vi "observacao.vi"() -> ()   [LabVIEW 2018, in "Shared_160.lvlib"] (continued)
            n314 = Select(t=FALSE, s=w274, f=w271) -> (s? t:f=w273:bool)
            n315 = case shown="False" w276 {
              frame False {
                w313 = 0
                n316 = property on="BtPointPrecess" class="Bool"("DisabledEnum"=w313) -> ()  [unwired: 2 in, 2 out]
                n317 = property on="BtPointObjClear" class="Bool"("DisabledEnum"=w313) -> ()  [unwired: 2 in, 2 out]
              }
              frame True {
                w314 = 2
                n318 = property on="BtPointPrecess" class="Bool"("DisabledEnum"=w314) -> ()  [unwired: 2 in, 2 out]
                n319 = property on="BtPointObjClear" class="Bool"("DisabledEnum"=w314) -> ()  [unwired: 2 in, 2 out]
              }
            }
            n320 = case shown="True" w273 {
              tunnel: [w384 w401] -> w299
              tunnel: [w383 w400] -> w295
              tunnel: [w386 w404] -> w275
              tunnel: [w385 w402] -> w292
              tunnel: w307 -> [w384 w401]
              tunnel: w306 -> [w389 _]
              tunnel: w305 -> [w388 _]
              tunnel: w302 -> [w387 _]
              tunnel: [w382 w398] -> _
              tunnel: w269 -> [w382 w398]
              frame False {
                n321 = case shown="True" w387 {
                  tunnel: w388 -> [w391 w397]
                  tunnel: [w391 w396] -> w386
                  tunnel: w389 -> [w390 w395]
                  tunnel: [w390 w392] -> w385
                  frame False {
                  }
                  frame True {
                    n322 = global read "Global_Telescopio.vi" "Calagem AH"() -> (w393:dbl)
                    n323 = global read "Global_Telescopio.vi" "Calagem DEC"() -> (w394:dbl)
                    n324 = Subtract(x=w395, y=w393) -> (x-y=w392:dbl)
                    n325 = Subtract(x=w397, y=w394) -> (x-y=w396:dbl)
                  }
                }
                n326 = Subtract(x=w384, y=w385) -> (x-y=w383:dbl)
              }
              frame True {
                # "PROCESSO PRECESSÃO"
                n327 = local read "Temp amb"() -> (w407:string)
                n328 = local read "hum local"() -> (w405:string)
                n329 = local read "MeanDEC"() -> (w408:string)
                n330 = local read "pressão atm"() -> (w406:string)
                n331 = local read "PM_RA"() -> (w403:string)
                n332 = local read "MeanRA"() -> (w409:string)
                n333 = local read "PM_DEC"() -> (w399:string)
                n334 = call "PrecessFortran.vi"("Asc reta"=w409, "Var RA"=w403, "Declinação"=w408, "Temperatura (Kelvin)"=w407, "Pressao atmosferica (mB)"=w406, "Humidade relativa (0 a 1)"=w405, "Var DEC"=w399) -> ("Observed RA (radians)"=w400:dbl, "Observed Dec (radians)"=w404:dbl)  [unwired: 2 in, 5 out]
                n335 = Subtract(x=w401, y=w400) -> (x-y=w402:dbl)
              }
            }
            "AtualDEC" <- w275
            n336 = case shown="True" w273 {
              tunnel: [w335 w338] -> w304
              tunnel: [w335 w337] -> w303
              tunnel: w275 -> [_ w336]
              frame False {
                w335 = 0.0
              }
              frame True {
                n337 = stacked-sequence {
                  seq-local: [w339 _ _] -> [_ _ w377]
                  tunnel: [_ w346 _] -> w338
                  tunnel: [_ w345 _] -> w337
                  tunnel: w336 -> [_ w340 _]
                  frame #0 {
                    n338 = Tick Count (ms)() -> (millisecond timer value=w339:u32)
                  }
                  frame #1 {
                    w347 = u16 3 items=["Alarme", "Atencao", "Erro", "Ocupado", "Protecao", "Embreagem", "Tracking", "Var. Track", "Rápido", "Ligeiro", "Médio", "Lento", "Em movimento", ""] ("NomeStatus")
                    w348 = u16 3 items=["Alarme", "Atencao", "Erro", "Ocupado", "Protecao", "Embreagem", "Tracking", "Var. Track", "Rápido", "Ligeiro", "Médio", "Lento", "Em movimento", ""] ("NomeStatus")
                    # "PROCESSO LEITURA POS_MOTOR"
                    n339 = local read "MOV_IDX_AH"() -> (w343:bool)
                    n340 = local read "MOV_IDX_DEC"() -> (w341:bool)
                    n341 = call "Bit Status AH.vi"("NomeStatus"=w348) -> ("StatBit"=w344:bool)
                    n342 = call "Bit Status DEC.vi"("NomeStatus"=w347) -> ("StatBit"=w342:bool)
                    n343 = case shown="False" w344 {
                      tunnel: w340 -> [w362 _]
                      tunnel: [w361 w376] -> w346
                      tunnel: w343 -> [w360 _]
                      frame False {
                        n344 = case shown="False" w360 {
                          tunnel: w362 -> [w370 _]
                          tunnel: [w366 w375] -> w361
                          frame False {
                            w373 = u16 1 items=["ZERO", "AH", "DEC", "TUBO", "CUP"] ("Controlador")
                            # "RA"
                            # "AH"
                            n345 = call "Get Posic Motor Indexer.vi"("Controlador"=w373) -> ("PosMotor"=w364:dbl)
                            n346 = global read "Global_Telescopio.vi" "AcumPrecRA"() -> (w367:dbl)
                            n347 = Negate(x=w364) -> (-x=w365:dbl)
                            n348 = Subtract(x=w365, y=w367) -> (x-y=w374:dbl)
                            n349 = global read "Global_Telescopio.vi" "AcumAG RA"() -> (w368:dbl)
                            n350 = Cosine(x=w370) -> (cos(x)=w369:dbl)
                            n351 = Absolute Value(x=w369) -> (abs(x)=w363:dbl)
                            n352 = Subtract(x=w374, y=w368) -> (x-y=w372:dbl)
                            n353 = Multiply(x=w363, y=w372) -> (x*y=w371:dbl)
                            n354 = call "Rad to Arcsec.vi"("Radiano"=w371) -> ("Arcsec"=w366:dbl)
                          }
                          frame True {
                            n355 = local read "Offset RA"() -> (w375:dbl)
                          }
                        }
                      }
                      frame True {
                        n356 = local read "Offset RA"() -> (w376:dbl)
                      }
                    }
                    n357 = case shown="False" w342 {
                      tunnel: [w350 w359] -> w345
                      tunnel: w341 -> [w349 _]
                      frame False {
                        n358 = case shown="False" w349 {
                          tunnel: [w351 w358] -> w350
                          frame False {
                            w354 = u16 2 items=["ZERO", "AH", "DEC", "TUBO", "CUP"] ("Controlador")
                            n359 = call "Get Posic Motor Indexer.vi"("Controlador"=w354) -> ("PosMotor"=w356:dbl)
                            n360 = global read "Global_Telescopio.vi" "AcumPrecDEC"() -> (w352:dbl)
                            n361 = Subtract(x=w356, y=w352) -> (x-y=w357:dbl)
                            n362 = global read "Global_Telescopio.vi" "AcumAG DEC"() -> (w353:dbl)
                            n363 = Subtract(x=w357, y=w353) -> (x-y=w355:dbl)
                            n364 = call "Rad to Arcsec.vi"("Radiano"=w355) -> ("Arcsec"=w351:dbl)
                          }
                          frame True {
                            n365 = local read "Offset DEC"() -> (w358:dbl)
                          }
                        }
                      }
                      frame True {
                        n366 = local read "Offset DEC"() -> (w359:dbl)
                      }
                    }
                  }
                  frame #2 {
                    n367 = flat-sequence {
                      tunnel: w377 -> [w378]
                      frame #0 {
                        n368 = Tick Count (ms)() -> (millisecond timer value=w379:u32)
                        n369 = Subtract(x=w379, y=w379) -> (x-y=→"dtAUX2":u32)
                        n370 = Subtract(x=w379, y=w378) -> (x-y=→"dtAUX3":u32)
                      }
                    }
                  }
                }
              }
            }
            "Offset RA" <- w304
            "Offset DEC" <- w303
            n371 = Add(x=w297, y=w295) -> (x+y=w296:dbl)
            n372 = Add(x=w297, y=w299) -> (x+y=w300:dbl)
            n373 = Less Than 0?(x=w299) -> (x < 0?=w301:bool)
            n374 = Less Than 0?(x=w295) -> (x < 0?=w298:bool)
            n375 = call "Normliza_AH.vi"("PosAH"=w292) -> ("Numeric"=w279:dbl)
            n376 = Select(t=w300, s=w301, f=w299) -> (s? t:f=w280:dbl)
            n377 = Select(t=w296, s=w298, f=w295) -> (s? t:f=w281:dbl)
            n378 = case shown="True" w271 {
              tunnel: ["" w322] -> w282
              tunnel: w281 -> [_ w319]
              tunnel: w280 -> [_ w320]
              tunnel: w275 -> [_ w321]
              frame False {
              }
              frame True {
                n379 = disable-structure shown="Disabled" {
                  disable-tunnel: w321 -> [w333 _]
                  disable-tunnel: w320 -> [w332 _]
                  disable-tunnel: w319 -> [w331 _]
                  disable-tunnel: [w330 _] -> _
                  frame Disabled {
                    n380 = call "Hora_Limite.vi"("Asc Reta RA rad"=w331, "Sideral Time rad"=w332, "Declinação rad"=w333) -> ("TO Tempo de Observação Horas"=w330:dbl)  [unwired: 2 in]
                  }
                  frame Enabled {
                  }
                }
                n381 = call "Novo_tempo_obs.vi"() -> ("TO rad"=w317:dbl)  [unwired: 10 in, 1 out]
                n382 = Greater Than 0?(x=w317) -> (x > 0?=w316:bool)
                n383 = case shown="True" w316 {
                  tunnel: [w324 w327] -> w318
                  tunnel: w317 -> [w324 w326]
                  frame False {
                  }
                  frame True {
                    n384 = Random Number (0-1)() -> (number: 0 to 1=w328:dbl)
                    n385 = Multiply(x=w328, y=7.27e-05) -> (x*y=w325:dbl)
                    n386 = Add(x=w326, y=w325) -> (x+y=w327:dbl)
                  }
                }
                n387 = call "rad_hms.vi"("TRUE=HORA\nFALSE=GRAU"=TRUE ("TRUE=HORA\nFALSE=GRAU"), "Radiano"=w318) -> ("Hora/Graus Texto Decimal"=w322:string)  [unwired: 3 in]
              }
            }
            "Time to Limit" <- w282
            n388 = global write "Global_Telescopio.vi" "AH_now"(w279) -> ()
            n389 = call "rad_hms.vi"("TRUE=HORA\nFALSE=GRAU"=TRUE ("TRUE=HORA\nFALSE=GRAU"), "Radiano"=w280) -> ("Hora/Graus Texto Decimal"=w294:string)  [unwired: 3 in]
            "Sideral time" <- w294
            n390 = call "rad_hms.vi"("TRUE=HORA\nFALSE=GRAU"=TRUE, "Radiano"=w281) -> ("Hora/Graus Texto Decimal"=w293:string)  [unwired: 3 in]
            "Right Ascention" <- w293
            n391 = call "rad_hms.vi"("TRUE=HORA\nFALSE=GRAU"=TRUE, "Radiano"=w279) -> ("Hora/Graus Texto Decimal"=w278:string)  [unwired: 3 in]
            "Hour Angle" <- w278
            "Hour Angle 2" <- w278
            n392 = call "rad_hms.vi"("TRUE=HORA\nFALSE=GRAU"=FALSE, "Radiano"=w275) -> ("Hora/Graus Texto Decimal"=w277:string)  [unwired: 3 in]
            "Declination" <- w277
            "DEC" <- w277
            n393 = global write "Global_Telescopio.vi" "Right Ascention"(w293) -> ()
            n394 = global write "Global_Telescopio.vi" "Hour Angle"(w278) -> ()
            n395 = global write "Global_Telescopio.vi" "Sideral time"(w294) -> ()
            n396 = global write "Global_Telescopio.vi" "Declination"(w277) -> ()
            n397 = global write "Global_Telescopio.vi" "delta_now"(w275) -> ()
          }
          frame #2 {
            w433 = -0.39330025  # LatOPD rad
            # "ALTERAÇÃO FEITA EM 12/12/2012\nFEITA PARA RESOLVER EXCESSÍVOS\nMOVIMENTOS DO ACOMP.SID. DA\nCÚPULA (DANIEL). A condição de statCUP=0 foi inserida em 08/5/2013-> Só corrige a cúpula se esta estiver parada!"
            # "Horas"
            # "MUDANÇA FUTURA:\nPassar LatOPD para Global"
            # "az"
            # "z"
            # "Cálculo do Azimute da Cúpula e Hab Acompanham. Cúpula"
            # "Lógica de Segurança"
            # "ANGULO ZENITAL"
            n398 = global read "Global_Telescopio.vi" "OffsetCupula"() -> (w442:dbl)
            n399 = global read "Global_Telescopio.vi" "AH_now"() -> (w425:dbl)
            n400 = global read "Global_Telescopio.vi" "delta_now"() -> (w432:dbl)
            n401 = global read "Global_Telescopio.vi" "Limite EAST"() -> (w426:dbl)
            n402 = global read "Global_Telescopio.vi" "Limite WEST"() -> (w427:dbl)
            n403 = call "Calculo_do_Azimute_da_Cupula_2.vi"("AH"=w425, "DEC"=w432, "OffsetTCSPD"=w442) -> ("PosCup"=w411:u16)  [unwired: 3 in, 1 out]
            "Azimute cup" <- w411
            n404 = local read "Tick Cupula"() -> (w417:u32)
            n405 = Tick Count (ms)() -> (millisecond timer value=w418:u32)
            n406 = global read "Global_Telescopio.vi" "PosCUP"() -> (→"PosCUP":i16)
            n407 = Multiply(x=w425, y=3.8197) -> (x*y=w428:dbl)
            n408 = call "Altura_e_Azimute.vi"("LAT rad"=w433, "DEC rad"=w432, "AH rad"=w425) -> ("AZIMUTE graus"=w413:dbl, "ANG. ZENITAL graus"=w431:dbl, "AZIMUTE rad"=w434:dbl, "ANG. ZENITAL rad"=w435:dbl)  [unwired: 2 out]
            "Azimuth" <- w413
            "Zenital angle" <- w431
            n409 = Greater Or Equal?(x=w418, y=w417) -> (x >= y?=w416:bool)
            n410 = Greater?(x=w428, y=w426) -> (0:w424:bool)
            n411 = Less?(x=w428, y=w427) -> (x < y?=w423:bool)
            n412 = call "Checa destino cupula.vi"("Target"=w411) -> ("moverCup"=w410:bool)  [unwired: 6 in, 2 out]
            n413 = local read "statCUP"() -> (w415:i32)
            n414 = Not And(1:w423, 2:w424) -> (0:w420:bool)
            n415 = Equal To 0?(x=w415) -> (x = 0?=w414:bool)
            n416 = call "Calcula_Proteção.vi"("Zenital angle rad"=w435, "Azimute rad"=w434) -> ("Z_SEGURANÇA_GRAUS"=w444:dbl, "Prot Segur"=w446:bool, "Z_LIBERA_GRAUS"=w443:dbl, "Z_MAX_GRAUS"=w445:dbl, "Prot Zmax"=w421:bool)
            n417 = Compound Arithmetic op=AND(w410, "DOME", w416, w414) -> (w441:bool)
            n418 = case shown="True" w441 {
              tunnel: w411 -> [_ w450]
              tunnel: FALSE -> [_ w455]
              frame False {
              }
              frame True {
                # "TEMPO CÚPULA"
                # "2m Tempo para novo movimento"
                n419 = Tick Count (ms)() -> (millisecond timer value=w454:u32)
                n420 = local write "Dome on Target"(w455) -> ()
                n421 = To Word Integer(number=w450) -> (16bit integer=w451:i16)
                n422 = Add(x=w454, y=u32 120000) -> (x+y=→"Tick Cupula":u32)
                n423 = local write "statCUP"(1 ("statCUP")) -> ()
                n424 = Number To Decimal String(number=w450) -> (decimal integer string=→"TargetCup":string)  [unwired: 1 in]
                n425 = global write "Global_Telescopio.vi" "TargetCUP"(w451) -> ()
              }
            }
            n426 = global write "Global_Telescopio.vi" "Z_SEGURANÇA_GRAUS"(w444) -> ()
            n427 = global write "Global_Telescopio.vi" "Zenital angle GRAUS"(w431) -> ()
            n428 = global write "Global_Telescopio.vi" "Azimute GRAUS"(w413) -> ()
            n429 = global write "Global_Telescopio.vi" "Z_MAX_GRAUS"(w445) -> ()
            n430 = global write "Global_Telescopio.vi" "Z_LIBERA_GRAUS"(w443) -> ()
            n431 = global read "Global_Telescopio.vi" "LIMITE"() -> (w440:bool)
            n432 = Or(x=w420, y=w421) -> (x .or. y?=w422:bool)
            n433 = Or(x=w440, y=w422) -> (x .or. y?=w439:bool)
            "Proteção" <- w439
            n434 = call "Borda_Subida_Z_max.vi"("Entrada"=w439) -> ("Boolean"=w448:bool)
            n435 = call "Borda_Subida_Segurança.vi"("Entrada"=w446) -> ("Boolean"=w447:bool)
            n436 = case shown="True" w448 {
              frame False {
              }
              frame True {
                w463 = FALSE
                w461 = "Telescópio parado por inclinação excessiva!" ("SYSTEM MESSAGES")
                n437 = local write "LED MOUNT"(w463) -> ()
                n438 = local write "MOUNT"(w463) -> ()
                n439 = global write "Global_Telescopio.vi" "ObjCentrado"(FALSE) -> ()
                n440 = global write "Global_Telescopio.vi" "STOP ALL"(TRUE ("STOP ALL")) -> ()
                n441 = call "Monta_Mensagem.vi"("Mensagem"=w461) -> ()  [unwired: 2 in]
                n442 = call "Salva_systems_messages.vi"("Mensagem"=w461) -> ()  [unwired: 5 in]
              }
            }
            n443 = Select(t=u8 2 ("Disabled"), s=w439, f=u8 0 ("Disabled")) -> (s? t:f=w436:u8)
            n444 = case shown="True" w447 {
              frame False {
              }
              frame True {
                w459 = u16 2 items=["ZERO", "AH", "DEC", "TUBO", "CUP"] ("Controlador")
                w458 = "FREAR" ("Comando")
                w460 = u16 1 items=["ZERO", "AH", "DEC", "TUBO", "CUP"] ("Controlador")
                w457 = "EIXO" ("Dispositivo")
                n445 = call "Monta Comando.vi"("Comando"=w458, "Dispositivo"=w457, "Controlador"=w460) -> ()  [unwired: 2 in, 5 out]
                n446 = call "Monta Comando.vi"("Comando"=w458, "Dispositivo"=w457, "Controlador"=w459) -> ()  [unwired: 2 in, 5 out]
              }
            }
            n447 = property on="MOUNT" class="Bool (strict)"("Disabled"=w436) -> ()  [unwired: 2 in, 2 out]
            "Led Chave Dome" <- "DOME"
          }
          frame #3 {
            w470 = u32 500 ("millisecond multiple")
            w484 = u16 3 items=["Alarme", "Atencao", "Erro", "Ocupado", "TBD", "LCB", "Trapeira", "Paravento", "DomoRap", "DomoCW", "DomoCCW", "TBD", "Em movimento", "TBD"] ("NomeStatus")
            w496 = u16 3 items=["Alarme", "Atencao", "Erro", "Ocupado", "Protecao", "Embreagem", "Tracking", "Var. Track", "Rápido", "Ligeiro", "Médio", "Lento", "Em movimento", ""] ("NomeStatus")
            w497 = u16 3 items=["Alarme", "Atencao", "Erro", "Ocupado", "Protecao", "Embreagem", "Tracking", "Var. Track", "Rápido", "Ligeiro", "Médio", "Lento", "Em movimento", ""] ("NomeStatus")
            # "04-07-2022\nValor de Erro PROTEC\nalterado de 5 para 10"
            # "MUDANÇA: \nIncluído CASE"
            # "Esse metrônomo determina\no ciclo de 0,5 segundo dos\ncálculos rápidos e totais!"
            # "PROCESSO APONTAMENTO"
            # "MÁQUINA DE ESTADO DO APONTAMENTO"
            # "Seta nome para GO/STOP"
            n448 = global read "Global_Telescopio.vi" "PosDEC"() -> (w499:dbl)
            n449 = global read "Global_Telescopio.vi" "TargetDEC"() -> (w500:dbl)
            n450 = global read "Global_Telescopio.vi" "LimiarRapMed"() -> (w498:dbl)
            n451 = global read "Global_Telescopio.vi" "ErroMaxEixo"() -> (w487:dbl)
            n452 = call "Bit Status DEC.vi"("NomeStatus"=w496) -> ("StatBit"=w486:bool)
            n453 = global read "Global_Telescopio.vi" "Sideral Time"() -> (w478:dbl)
            n454 = global read "Global_Telescopio.vi" "PosAH"() -> (w501:dbl)
            n455 = global read "Global_Telescopio.vi" "TargetRA"() -> (w502:dbl)
            n456 = global write "Global_Telescopio.vi" "Estado AH"("statAH") -> ()
            n457 = call "Bit Status AH.vi"("NomeStatus"=w497) -> ("StatBit"=w485:bool)
            n458 = case shown="40" "statDEC" {
              selector: "statDEC" -> [w631 _ _ _ _ _ _ _ _]
              tunnel: [w631 w638 w668 w690 w717 w741 0 ("t") w758 w768] -> w479
              tunnel: w500 -> [_ w637 _ w684 _ _ _ _ w774]
              tunnel: w499 -> [_ w633 _ w687 _ _ _ _ w773]
              tunnel: w487 -> [_ _ _ w688 _ _ _ _ w771]
              tunnel: w498 -> [_ w639 _ _ _ _ _ _ _]
              tunnel: w486 -> [_ w636 _ w683 _ _ _ _ _]
              frame 0, Default {
                w629 = 0 ("CR DEC")
                # "Sem apontamento"
                n459 = call "TickTimeout.vi"() -> ("msTick"=→"TimeoutDEC":u32)  [unwired: 2 in, 2 out]
                n460 = local write "CR DEC"(w629) -> ()
                n461 = local write "C. DEC"(w629) -> ()
              }
              frame 1 {
                # "Envia\nComando"
                n462 = Subtract(x=w637, y=w633) -> (x-y=w635:dbl)
                n463 = Absolute Value(x=w635) -> (abs(x)=w640:dbl)
                n464 = local write "dec="(FALSE ("dec=")) -> ()
                n465 = Less?(x=w640, y=w639) -> (x < y?=w634:bool)
                n466 = case shown="False" w634 {
                  tunnel: [w644 3] -> w638
                  tunnel: w637 -> [w643 _]
                  tunnel: w635 -> [w642 _]
                  tunnel: w636 -> [w641 _]
                  frame False {
                    # "destino"
                    # "Fora do"
                    n467 = case shown="False" w641 {
                      tunnel: [w648 w656] -> w644
                      tunnel: w643 -> [w651 _]
                      tunnel: w642 -> [_ _]
                      frame False {
                        w655 = u16 2 items=["ZERO", "AH", "DEC", "TUBO", "CUP"] ("Controlador")
                        # "limpa flag"
                        # "CLP Pronto"
                        n468 = local write "Flag ativo DEC"(FALSE ("Flag ativo DEC")) -> ()
                        n469 = call "rad_hms.vi"("TRUE=HORA\nFALSE=GRAU"=FALSE, "Radiano"=w651) -> ("Hora/Graus Texto Decimal"=w652:string)  [unwired: 3 in]
                        n470 = call "Monta Comando.vi"("Set Point"=w652, "Comando"="MOVER_RAP", "Dispositivo"="EIXO" ("Comando"), "Controlador"=w655) -> ("Erro Comunicação"=w646:bool)  [unwired: 1 in, 4 out]
                        n471 = Select(t=6, s=w646, f=20) -> (s? t:f=w648:i32)
                      }
                      frame True {
                        # "CLP Ocupado"
                        n472 = local read "TimeoutDEC"() -> (w658:u32)
                        n473 = call "TickTimeout.vi"("msInicial"=w658, "msTimeout"=u32 4000) -> ("Timeout"=w657:bool)  [unwired: 2 out]
                        n474 = case shown="False" w657 {
                          tunnel: [1 5] -> w656
                          frame False {
                          }
                          frame True {
                            # "Tratar\nTimeout"
                          }
                        }
                      }
                    }
                  }
                  frame True {
                    # "Dist. pequena p/ mov. rápido"
                    # "Ligar mov. lento"
                    n475 = call "TickTimeout.vi"() -> ("msTick"=w662:u32)  [unwired: 2 in, 2 out]
                    n476 = local write "TimeoutDEC"(w662) -> ()
                  }
                }
              }
              frame 2 {
                w669 = u16 12 items=["Alarme", "Atencao", "Erro", "Ocupado", "Protecao", "Embreagem", "Tracking", "Var. Track", "Rápido", "Ligeiro", "Médio", "Lento", "Em movimento", ""] ("NomeStatus")
                # "Aguarda fim mov. Rap."
                n477 = global read "Global_Telescopio.vi" "Habilita supervisao"() -> (w665:bool)
                n478 = call "Bit Status DEC.vi"("NomeStatus"=w669) -> ("StatBit"=w670:bool)
                n479 = case shown="True" w670 {
                  tunnel: [1 w679] -> w667
                  frame False {
                    # "Motor parado.\nTestar se chegou\nao destino"
                    n480 = call "TickTimeout.vi"() -> ("msTick"=w675:u32)  [unwired: 2 in, 2 out]
                    n481 = local write "TimeoutDEC"(w675) -> ()
                  }
                  frame True {
                    # "Ainda movendo...\nAGUARDAR"
                    n482 = local read "Erro PROTEC"() -> (w681:i32)
                    n483 = call "PROTECAO_DEC.vi"() -> ("CONT DEC"=w682:i32)  [unwired: 11 in]
                    "C. DEC" <- w682
                    n484 = Greater Or Equal?(x=w682, y=w681) -> (x >= y?=w677:bool)
                    n485 = Select(t=6, s=w677, f=2) -> (s? t:f=w679:i32)
                  }
                }
                n486 = case shown="False" w665 {
                  tunnel: [FALSE w674] -> w664
                  frame False {
                  }
                  frame True {
                    n487 = local read "Erro Lim"() -> (w672:i32)
                    n488 = Greater Or Equal?(x="CR DEC", y=w672) -> (x >= y?=w674:bool)
                  }
                }
                n489 = Select(t=6, s=w664, f=w667) -> (s? t:f=w668:i32)
              }
              frame 3 {
                # "Mov.Lento"
                n490 = Subtract(x=w684, y=w687) -> (x-y=w685:dbl)
                n491 = Absolute Value(x=w685) -> (abs(x)=w689:dbl)
                n492 = Less Or Equal?(x=w689, y=w688) -> (x <= y?=w686:bool)
                n493 = case shown="False" w686 {
                  selector: w686 -> [_ w713]
                  tunnel: [w692 0] -> w690
                  tunnel: w685 -> [w691 _]
                  tunnel: w684 -> [_ w712]
                  tunnel: w683 -> [w693 _]
                  frame False {
                    n494 = case shown="False" w693 {
                      tunnel: [w697 w706] -> w692
                      tunnel: w691 -> [w700 _]
                      frame False {
                        w705 = u16 2 items=["ZERO", "AH", "DEC", "TUBO", "CUP"] ("Controlador")
                        # "limpa flag"
                        # "Mov. lento"
                        n495 = call "rad_hms.vi"("TRUE=HORA\nFALSE=GRAU"=FALSE ("TRUE=HORA\nFALSE=GRAU"), "Radiano"=w700) -> ("Hora/Graus Texto Decimal"=w702:string)  [unwired: 3 in]
                        n496 = call "Monta Comando.vi"("Set Point"=w702, "Comando"="MOVER_REL", "Dispositivo"="EIXO" ("Comando"), "Controlador"=w705) -> ("Erro Comunicação"=w695:bool)  [unwired: 1 in, 4 out]
                        n497 = call "TickTimeout.vi"() -> ("msTick"=w699:u32)  [unwired: 2 in, 2 out]
                        n498 = local write "Flag ativo DEC"(FALSE ("Flag ativo DEC")) -> ()
                        n499 = local write "TimeoutDEC"(w699) -> ()
                        n500 = Select(t=6, s=w695, f=40) -> (s? t:f=w697:i32)
                      }
                      frame True {
                        # "CLP Ocupado"
                        n501 = local read "TimeoutDEC"() -> (w708:u32)
                        n502 = call "TickTimeout.vi"("msInicial"=w708, "msTimeout"=u32 2000) -> ("Timeout"=w707:bool)  [unwired: 2 out]
                        n503 = case shown="False" w707 {
                          tunnel: [3 5] -> w706
                          frame False {
                          }
                          frame True {
                          }
                        }
                      }
                    }
                  }
                  frame True {
                    # "DEC no destino"
                    n504 = local write "LatchDeslocDEC"(w712) -> ()
                    "DEC on Target" <- w713
                  }
                }
              }
              frame 4 {
                w720 = u16 12 items=["Alarme", "Atencao", "Erro", "Ocupado", "Protecao", "Embreagem", "Tracking", "Var. Track", "Rápido", "Ligeiro", "Médio", "Lento", "Em movimento", ""] ("NomeStatus")
                # "Aguarda fim mov. lento"
                n505 = global read "Global_Telescopio.vi" "Habilita supervisao"() -> (w718:bool)
                n506 = call "Bit Status DEC.vi"("NomeStatus"=w720) -> ("StatBit"=w721:bool)
                n507 = case shown="False" w721 {
                  tunnel: [3 w731] -> w716
                  frame False {
                    # "Motor parado.\nTestar se chegou\nao destino"
                    n508 = call "TickTimeout.vi"() -> ("msTick"=w726:u32)  [unwired: 2 in, 2 out]
                    n509 = local write "TimeoutDEC"(w726) -> ()
                  }
                  frame True {
                    n510 = local read "Erro PROTEC"() -> (w733:i32)
                    n511 = call "PROTECAO_DEC.vi"() -> ("CONT DEC"=w728:i32)  [unwired: 11 in]
                    n512 = local write "C. DEC"(w728) -> ()
                    n513 = Greater Or Equal?(x=w728, y=w733) -> (x >= y?=w730:bool)
                    n514 = local read "TimeoutDEC"() -> (w735:u32)
                    n515 = call "TickTimeout.vi"("msInicial"=w735, "msTimeout"=u32 4000) -> ("Timeout"=w734:bool)  [unwired: 2 out]
                    n516 = case shown="False" w734 {
                      tunnel: [4 5] -> w729
                      frame False {
                      }
                      frame True {
                      }
                    }
                    n517 = Select(t=6, s=w730, f=w729) -> (s? t:f=w731:i32)
                  }
                }
                n518 = case shown="True" w718 {
                  tunnel: [FALSE w725] -> w715
                  frame False {
                  }
                  frame True {
                    n519 = local read "CR DEC"() -> (w724:i32)
                    n520 = local read "Erro Lim"() -> (w723:i32)
                    n521 = Greater Or Equal?(x=w724, y=w723) -> (x >= y?=w725:bool)
                  }
                }
                n522 = Select(t=6, s=w715, f=w716) -> (s? t:f=w717:i32)
              }
              frame 5 {
                w746 = u16 2 items=["ZERO", "AH", "DEC", "TUBO", "CUP"] ("Controlador")
                # "Reiniciar apontamento"
                # "Trata Timeout"
                n523 = call "TickTimeout.vi"() -> ("msTick"=w743:u32)  [unwired: 2 in, 2 out]
                n524 = local write "TimeoutDEC"(w743) -> ()
                n525 = call "Monta Comando.vi"("Comando"="PARAR", "Dispositivo"="PROG" ("Comando"), "Controlador"=w746) -> ("Erro Comunicação"=w739:bool)  [unwired: 2 in, 4 out]
                n526 = Select(t=6, s=w739, f=1) -> (s? t:f=w741:i32)
              }
              frame 6 {
                # "PARADA POR ERRO DO CONTROLADOR"
                n527 = stacked-sequence {
                  frame #0 {
                    w749 = u16 2 items=["ZERO", "AH", "DEC", "TUBO", "CUP"] ("Controlador")
                    n528 = call "Monta Comando.vi"("Comando"="PARAR", "Dispositivo"="PROG" ("Comando"), "Controlador"=w749) -> ()  [unwired: 2 in, 5 out]
                    "dec=" <- TRUE ("ah=")
                  }
                  frame #1 {
                    w752 = "Erro de Controlador DEC , REAPONTAR !" ("Mensagem")
                    n529 = local write "Flag de erro p/ apagar lampada"(TRUE ("Flag de erro p/ apagar lampada")) -> ()
                    n530 = call "Monta_Mensagem.vi"("Mensagem"=w752) -> ()  [unwired: 2 in]
                    n531 = call "Salva_systems_messages.vi"("Mensagem"=w752) -> ()  [unwired: 5 in]
                  }
                  frame #2 {
                    w755 = u16 2 items=["ZERO", "AH", "DEC", "TUBO", "CUP"] ("Controlador")
                    # "Em movimento não aceita reset"
                    # "Segundo PARAR por garantia"
                    n532 = call "Monta Comando.vi"("Comando"="PARAR", "Dispositivo"="PROG", "Controlador"=w755) -> ()  [unwired: 2 in, 5 out]
                  }
                }
              }
              frame 20 {
                # "Espera entrar\nem movimento"
                n533 = local read "Flag ativo DEC"() -> (w757:bool)
                n534 = case shown="True" w757 {
                  tunnel: [20 ("t") 2 ("t")] -> w758
                  frame False {
                  }
                  frame True {
                    # "limpa flag"
                    n535 = local write "Flag ativo DEC"(FALSE ("Flag ativo AH")) -> ()
                  }
                }
              }
              frame 40 {
                # "INTERROMPE O\nMOVIMENTO"
                # "Espera entrar\nem movimento"
                n536 = Subtract(x=w774, y=w773) -> (x-y=w772:dbl)
                n537 = Absolute Value(x=w772) -> (abs(x)=w775:dbl)
                n538 = Less Or Equal?(x=w775, y=w771) -> (x <= y?=w763:bool)
                n539 = local read "Flag ativo DEC"() -> (w770:bool)
                n540 = local read "TimeoutDEC"() -> (w766:u32)
                n541 = call "TickTimeout.vi"("msInicial"=w766, "msTimeout"=u32 25000) -> ("Timeout"=w764:bool)  [unwired: 2 out]
                n542 = case shown="True" w770 {
                  tunnel: [40 ("t") 4 ("t")] -> w769
                  frame False {
                  }
                  frame True {
                    # "limpa flag"
                    n543 = local write "Flag ativo DEC"(FALSE ("Flag ativo AH")) -> ()
                  }
                }
                n544 = Or(x=w764, y=w763) -> (x .or. y?=w762:bool)
                n545 = Select(t=5, s=w762, f=w769) -> (s? t:f=w768:i32)
              }
            }
            n546 = global write "Global_Telescopio.vi" "Estado DEC"("statDEC") -> ()
            n547 = case shown="5" "statAH" {
              selector: "statAH" -> [w781 _ _ _ _ _ _ _ _ _]
              tunnel: [w781 w790 w818 w834 w858 w886 w911 0 ("t") w927 w932] -> w483
              tunnel: w478 -> [_ w787 _ _ w855 _ _ _ _ _]
              tunnel: w502 -> [_ w786 _ _ w852 _ _ _ _ _]
              tunnel: w501 -> [_ w784 _ _ w854 _ _ _ _ _]
              tunnel: w487 -> [_ _ _ _ w859 _ _ _ _ _]
              tunnel: w498 -> [_ w791 _ _ _ _ _ _ _ _]
              tunnel: w485 -> [_ w788 _ w835 w856 _ _ _ _ _]
              frame 0, Default {
                w779 = 0 ("CR AH")
                # "Sem apontamento"
                n548 = call "TickTimeout.vi"() -> ("msTick"=→"TimeoutAH":u32)  [unwired: 2 in, 2 out]
                n549 = local write "CR AH"(w779) -> ()
                n550 = local write "C. AH"(w779) -> ()
              }
              frame 1 {
                # "Mov.Rapido"
                n551 = call "Calculo_AH.vi"("AH_Telescopio"=w784, "RA_Destino"=w786, "Hora Sideral"=w787) -> ("Dif_Abs_AH"=w785:dbl, "AH_Destino"=w782:dbl)  [unwired: 1 out]
                "AH_Destino" <- w782
                n552 = Less?(x=w785, y=w791) -> (x < y?=w789:bool)
                n553 = case shown="False" w789 {
                  tunnel: w782 -> [w792 _]
                  tunnel: [w793 3] -> w790
                  tunnel: w788 -> [w794 _]
                  frame False {
                    n554 = case shown="True" w794 {
                      tunnel: w792 -> [w800 _]
                      tunnel: [w797 w806] -> w793
                      frame False {
                        w802 = u16 1 items=["ZERO", "AH", "DEC", "TUBO", "CUP"] ("Controlador")
                        # "limpa flag"
                        # "Aguardar\nfim mov."
                        # "Mov. rápido"
                        n555 = local write "Flag ativo AH"(FALSE ("Flag ativo AH")) -> ()
                        n556 = call "rad_hms.vi"("TRUE=HORA\nFALSE=GRAU"=TRUE ("TRUE=HORA\nFALSE=GRAU"), "Radiano"=w800) -> ("Hora/Graus Texto Decimal"=w805:string)  [unwired: 3 in]
                        n557 = call "Monta Comando.vi"("Set Point"=w805, "Comando"="MOVER_RAP", "Dispositivo"="EIXO" ("Comando"), "Controlador"=w802) -> ("Erro Comunicação"=w799:bool)  [unwired: 1 in, 4 out]
                        n558 = Select(t=7, s=w799, f=20) -> (s? t:f=w797:i32)
                      }
                      frame True {
                        # "CLP Ocupado"
                        n559 = local read "TimeoutAH"() -> (w808:u32)
                        n560 = call "TickTimeout.vi"("msInicial"=w808, "msTimeout"=u32 8000) -> ("Timeout"=w807:bool)  [unwired: 2 out]
                        n561 = case shown="True" w807 {
                          tunnel: [1 6] -> w806
                          frame False {
                          }
                          frame True {
                            # "Tratar\nTimeout"
                          }
                        }
                      }
                    }
                  }
                  frame True {
                    # "Ligar acomp. sideral"
                    # "Dist. pequena p/ mov. rápido"
                    n562 = call "TickTimeout.vi"() -> ("msTick"=w812:u32)  [unwired: 2 in, 2 out]
                    n563 = local write "TimeoutAH"(w812) -> ()
                  }
                }
                n564 = local write "ah="(FALSE ("ah=")) -> ()
              }
              frame 2 {
                w820 = u16 12 items=["Alarme", "Atencao", "Erro", "Ocupado", "Protecao", "Embreagem", "Tracking", "Var. Track", "Rápido", "Ligeiro", "Médio", "Lento", "Em movimento", ""] ("NomeStatus")
                # "Aguarda fim mov. Rap."
                n565 = call "Bit Status AH.vi"("NomeStatus"=w820) -> ("StatBit"=w819:bool)
                n566 = case shown="True" w819 {
                  tunnel: [1 w829] -> w817
                  frame False {
                    # "Motor parado.\nTestar se precisa\nde novo cmd. \nde mov. rápido"
                    n567 = call "TickTimeout.vi"() -> ("msTick"=w825:u32)  [unwired: 2 in, 2 out]
                    n568 = local write "TimeoutAH"(w825) -> ()
                  }
                  frame True {
                    # "Aqui também \ncaberia um \nTimeout?"
                    # "Ainda movendo...\nAGUARDAR"
                    n569 = local read "AH_Destino"() -> (w827:dbl)
                    n570 = local read "Erro PROTEC"() -> (w833:i32)
                    n571 = call "PROTECAO_AH.vi"("AH_Destino"=w827) -> ("CONT AH"=w828:i32)  [unwired: 10 in]
                    "C. AH" <- w828
                    n572 = Greater Or Equal?(x=w828, y=w833) -> (x >= y?=w832:bool)
                    n573 = Select(t=7, s=w832, f=2) -> (s? t:f=w829:i32)
                  }
                }
                n574 = global read "Global_Telescopio.vi" "Habilita supervisao"() -> (w815:bool)
                n575 = case shown="True" w815 {
                  tunnel: [FALSE w823] -> w814
                  frame False {
                  }
                  frame True {
                    n576 = local read "Erro Lim"() -> (w822:i32)
                    n577 = Greater Or Equal?(x="CR AH", y=w822) -> (x >= y?=w823:bool)
                  }
                }
                n578 = Select(t=7, s=w814, f=w817) -> (s? t:f=w818:i32)
              }
              frame 3 {
                # "Liga Acomp. Sideral"
                n579 = case shown="True" w835 {
                  tunnel: [w836 w845] -> w834
                  frame False {
                    w840 = TRUE
                    w842 = u16 1 items=["ZERO", "AH", "DEC", "TUBO", "CUP"] ("Controlador")
                    # "Usar mov. lento"
                    # "CLP Pronto - Liga sideral"
                    n580 = call "Monta Comando.vi"("Comando"="LIGAR", "Dispositivo"="SIDERAL" ("Comando"), "Controlador"=w842) -> ("Erro Comunicação"=w838:bool)  [unwired: 2 in, 4 out]
                    n581 = Select(t=7, s=w838, f=4) -> (s? t:f=w836:i32)
                    n582 = call "TickTimeout.vi"() -> ("msTick"=w841:u32)  [unwired: 2 in, 2 out]
                    n583 = local write "LED MOUNT"(w840) -> ()
                    n584 = local write "MOUNT"(w840) -> ()
                    n585 = local write "TimeoutAH"(w841) -> ()
                  }
                  frame True {
                    # "CLP Ocupado"
                    n586 = local read "TimeoutAH"() -> (w847:u32)
                    n587 = call "TickTimeout.vi"("msInicial"=w847, "msTimeout"=u32 8000) -> ("Timeout"=w846:bool)  [unwired: 2 out]
                    n588 = case shown="True" w846 {
                      tunnel: [3 6] -> w845
                      frame False {
                      }
                      frame True {
                        # "Tratar\nTimeout"
                      }
                    }
                  }
                }
              }
              frame 4 {
                # "Mov.Lento"
                n589 = call "Calculo_AH.vi"("AH_Telescopio"=w854, "RA_Destino"=w852, "Hora Sideral"=w855) -> ("Dif_AH"=w851:dbl, "Dif_Abs_AH"=w853:dbl)  [unwired: 1 out]
                n590 = Less?(x=w853, y=w859) -> (x < y?=w857:bool)
                n591 = case shown="True" w857 {
                  selector: w857 -> [_ w882]
                  tunnel: [w861 0] -> w858
                  tunnel: w856 -> [w862 _]
                  tunnel: w852 -> [_ w881]
                  tunnel: w851 -> [w860 _]
                  frame False {
                    n592 = case shown="True" w862 {
                      tunnel: [w865 w875] -> w861
                      tunnel: w860 -> [w869 _]
                      frame False {
                        w871 = u16 1 items=["ZERO", "AH", "DEC", "TUBO", "CUP"] ("Controlador")
                        # "limpa flag"
                        # "Envia Cmd. Mov. Lento"
                        n593 = call "TickTimeout.vi"() -> ("msTick"=w868:u32)  [unwired: 2 in, 2 out]
                        n594 = local write "TimeoutAH"(w868) -> ()
                        n595 = local write "Flag ativo AH"(FALSE ("Flag ativo AH")) -> ()
                        n596 = call "rad_hms.vi"("TRUE=HORA\nFALSE=GRAU"=TRUE ("TRUE=HORA\nFALSE=GRAU"), "Radiano"=w869) -> ("Hora/Graus Texto Decimal"=w874:string)  [unwired: 3 in]
                        n597 = call "Monta Comando.vi"("Set Point"=w874, "Comando"="MOVER_REL", "Dispositivo"="EIXO" ("Comando"), "Controlador"=w871) -> ("Erro Comunicação"=w864:bool)  [unwired: 1 in, 4 out]
                        n598 = Select(t=7, s=w864, f=50) -> (s? t:f=w865:i32)
                      }
                      frame True {
                        # "CLP Ocupado"
                        n599 = local read "TimeoutAH"() -> (w877:u32)
                        n600 = call "TickTimeout.vi"("msInicial"=w877, "msTimeout"=u32 8000) -> ("Timeout"=w876:bool)  [unwired: 2 out]
                        n601 = case shown="False" w876 {
                          tunnel: [4 6] -> w875
                          frame False {
                          }
                          frame True {
                          }
                        }
                      }
                    }
                  }
                  frame True {
                    # "AH on Target"
                    n602 = local write "LatchDeslocRA"(w881) -> ()
                    "RA on Target" <- w882
                  }
                }
              }
              frame 5 {
                w890 = u16 12 items=["Alarme", "Atencao", "Erro", "Ocupado", "Protecao", "Embreagem", "Tracking", "Var. Track", "Rápido", "Ligeiro", "Médio", "Lento", "Em movimento", ""] ("NomeStatus")
                # "Aguarda fim mov. Lento"
                n603 = call "Bit Status AH.vi"("NomeStatus"=w890) -> ("StatBit"=w889:bool)
                n604 = case shown="True" w889 {
                  tunnel: [4 w902] -> w884
                  frame False {
                    # "Motor parado.\nTestar se chegou\nao destino"
                    n605 = call "TickTimeout.vi"() -> ("msTick"=w895:u32)  [unwired: 2 in, 2 out]
                    n606 = local write "TimeoutAH"(w895) -> ()
                  }
                  frame True {
                    # "Trata Timeout"
                    n607 = local read "AH_Destino"() -> (w897:dbl)
                    n608 = local read "Erro PROTEC"() -> (w900:i32)
                    n609 = call "PROTECAO_AH.vi"("AH_Destino"=w897) -> ("CONT AH"=w898:i32)  [unwired: 10 in]
                    n610 = local read "TimeoutAH"() -> (w905:u32)
                    n611 = Greater Or Equal?(x=w898, y=w900) -> (x >= y?=w899:bool)
                    n612 = local write "C. AH"(w898) -> ()
                    n613 = call "TickTimeout.vi"("msInicial"=w905, "msTimeout"=u32 8000) -> ("Timeout"=w904:bool)  [unwired: 2 out]
                    n614 = case shown="False" w904 {
                      tunnel: [5 6] -> w901
                      frame False {
                      }
                      frame True {
                        # "Tratar\nTimeout"
                      }
                    }
                    n615 = Select(t=7, s=w899, f=w901) -> (s? t:f=w902:i32)
                  }
                }
                n616 = global read "Global_Telescopio.vi" "Habilita supervisao"() -> (w888:bool)
                n617 = case shown="True" w888 {
                  tunnel: [FALSE w894] -> w885
                  frame False {
                  }
                  frame True {
                    n618 = local read "Erro Lim"() -> (w892:i32)
                    n619 = local read "CR AH"() -> (w893:i32)
                    n620 = Greater Or Equal?(x=w893, y=w892) -> (x >= y?=w894:bool)
                  }
                }
                n621 = Select(t=7, s=w885, f=w884) -> (s? t:f=w886:i32)
              }
              frame 6 {
                w914 = u16 1 items=["ZERO", "AH", "DEC", "TUBO", "CUP"] ("Controlador")
                # "Reiniciar apontamento"
                # "Trata Timeout"
                n622 = call "TickTimeout.vi"() -> ("msTick"=w913:u32)  [unwired: 2 in, 2 out]
                n623 = call "Monta Comando.vi"("Comando"="PARAR", "Dispositivo"="PROG" ("Comando"), "Controlador"=w914) -> ("Erro Comunicação"=w909:bool)  [unwired: 2 in, 4 out]
                n624 = local write "TimeoutAH"(w913) -> ()
                n625 = Select(t=7, s=w909, f=1) -> (s? t:f=w911:i32)
              }
              frame 7 {
                # "PARADA POR ERRO DO CONTROLADOR"
                n626 = stacked-sequence {
                  frame #0 {
                    w919 = u16 1 items=["ZERO", "AH", "DEC", "TUBO", "CUP"] ("Controlador")
                    n627 = call "Monta Comando.vi"("Comando"="PARAR", "Dispositivo"="PROG" ("Comando"), "Controlador"=w919) -> ()  [unwired: 2 in, 5 out]
                    "ah=" <- TRUE ("ah=")
                  }
                  frame #1 {
                    w922 = "Erro de Controlador RA , REAPONTAR !" ("Mensagem")
                    n628 = call "Monta_Mensagem.vi"("Mensagem"=w922) -> ()  [unwired: 2 in]
                    n629 = call "Salva_systems_messages.vi"("Mensagem"=w922) -> ()  [unwired: 5 in]
                    "Flag de erro p/ apagar lampada" <- TRUE ("Flag de erro p/ apagar lampada")
                  }
                  frame #2 {
                    w926 = u16 1 items=["ZERO", "AH", "DEC", "TUBO", "CUP"] ("Controlador")
                    # "Em movimento não aceita reset"
                    # "Segundo PARAR por garantia"
                    n630 = call "Monta Comando.vi"("Comando"="PARAR", "Dispositivo"="PROG", "Controlador"=w926) -> ()  [unwired: 2 in, 5 out]
                  }
                }
              }
              frame 20 {
                # "Espera entrar\nem movimento"
                n631 = local read "Flag ativo AH"() -> (w928:bool)
                n632 = case shown="True" w928 {
                  tunnel: [20 ("t") 2 ("t")] -> w927
                  frame False {
                  }
                  frame True {
                    # "limpa flag"
                    n633 = local write "Flag ativo AH"(FALSE ("Flag ativo AH")) -> ()
                  }
                }
              }
              frame 50 {
                # "Espera entrar\nem movimento"
                n634 = local read "Flag ativo AH"() -> (w933:bool)
                n635 = case shown="True" w933 {
                  tunnel: [50 ("t") 5 ("t")] -> w932
                  frame False {
                  }
                  frame True {
                    # "limpa flag"
                    n636 = local write "Flag ativo AH"(FALSE ("Flag ativo AH")) -> ()
                  }
                }
              }
            }
            n637 = call "PROTECAO.vi"("Estado In"=w483) -> ("Estado Out"=w482:i32)  [unwired: 2 in]
            n638 = local write "statAH"(w482) -> ()
            n639 = local read "statCUP"() -> (w489:i32)
            n640 = local read "statDEC"() -> (w490:i32)
            n641 = call "PROTECAO.vi"("Estado In"=w479) -> ("Estado Out"=w465:i32)  [unwired: 2 in]
            n642 = global read "Global_Telescopio.vi" "TargetCUP"() -> (w494:i16)
            n643 = local read "statAH"() -> (w491:i32)
            n644 = global write "Global_Telescopio.vi" "Estado CUP"("statCUP") -> ()
            n645 = global read "Global_Telescopio.vi" "Botão GO = STOP"() -> (w477:bool)
            n646 = local write "statDEC"(w465) -> ()
            n647 = call "Bit Status CUP.vi"("NomeStatus"=w484) -> ("StatBit"=w495:bool)
            n648 = Compound Arithmetic op=ADD(w489, w491, w490) -> (w493:i32)
            n649 = case shown="1" "statCUP" {
              selector: "statCUP" -> [w514 _ _ _ _ _ _ _]
              tunnel: [w514 w522 w566 1 w576 w597 w606 w624] -> w481
              tunnel: w495 -> [_ w523 _ _ w578 _ w603 _]
              tunnel: w494 -> [_ w518 _ _ _ _ _ _]
              frame 0, Default {
                # "Sem movimento"
                n650 = call "TickTimeout.vi"() -> ("msTick"=→"TimeoutCUP":u32)  [unwired: 2 in, 2 out]
              }
              frame 1 {
                # "20240820"
                # "Envia\nComando"
                n651 = local read "LedPointing"() -> (w519:bool)
                n652 = local read "DOME"() -> (w520:bool)
                n653 = call "Checa destino cupula.vi"("Target"=w518) -> ("moverCup"=w516:bool, "angTarget"=w515:string)  [unwired: 6 in, 1 out]
                n654 = Not(x=w516) -> (.not. x?=w517:bool)
                n655 = case shown="False" w517 {
                  tunnel: w523 -> [w530 w556]
                  tunnel: w518 -> [w529 _]
                  tunnel: [w528 w557] -> w522
                  tunnel: "ChkDomeEnable" -> [w525 w555]
                  tunnel: w520 -> [w527 w554]
                  tunnel: w519 -> [w526 w553]
                  tunnel: w515 -> [w524 _]
                  frame False {
                    # "CUP fora pos."
                    n656 = case shown="False" w530 {
                      tunnel: w529 -> [w538 _]
                      tunnel: [w536 w547] -> w528
                      tunnel: w527 -> [w535 _]
                      tunnel: w526 -> [w533 _]
                      tunnel: w525 -> [w532 _]
                      tunnel: w524 -> [w531 _]
                      frame False {
                        # "CLP Pronto"
                        n657 = Number To Decimal String(number=w538) -> (decimal integer string=w537:string)  [unwired: 1 in]
                        n658 = Select(t=w532, s=w533, f=w535) -> (s? t:f=w534:bool)
                        n659 = case shown="True" w534 {
                          tunnel: [0 2] -> w536
                          tunnel: w537 -> [_ w541]
                          tunnel: w531 -> [_ w540]
                          frame False {
                            # "Cúpula Desabilitada"
                            # "Também não verifica\nTrapeira e Paravento"
                          }
                          frame True {
                            w545 = u16 4 items=["ZERO", "AH", "DEC", "TUBO", "CUP"] ("Controlador")
                            n660 = call "TickTimeout.vi"() -> ("msTick"=w543:u32)  [unwired: 2 in, 2 out]
                            n661 = local write "TargetCup"(w540) -> ()
                            n662 = local write "TimeoutCUP"(w543) -> ()
                            n663 = global write "Global_Telescopio.vi" "T cup"(w543) -> ()
                            n664 = call "Monta Comando.vi"("Set Point"=w541, "Comando"="MOVER", "Dispositivo"="DOMO" ("Comando"), "Controlador"=w545) -> ()  [unwired: 1 in, 5 out]
                          }
                        }
                      }
                      frame True {
                        # "CLP Busy"
                        n665 = local read "TimeoutCUP"() -> (w549:u32)
                        n666 = call "TickTimeout.vi"("msInicial"=w549, "msTimeout"=u32 5000) -> ("Timeout"=w548:bool)  [unwired: 2 out]
                        n667 = case shown="False" w548 {
                          tunnel: [1 3] -> w547
                          frame False {
                          }
                          frame True {
                          }
                        }
                      }
                    }
                  }
                  frame True {
                    # "CUP no destino"
                    n668 = case shown="True" w553 {
                      tunnel: [0 w561] -> w557
                      tunnel: w556 -> [_ _]
                      tunnel: w555 -> [_ w560]
                      tunnel: w554 -> [w558 _]
                      frame False {
                        # "Não está apontando (chave Dome Enable foi ativada)"
                        # "Não verifica\nTrapeira e\nParavento"
                        n669 = local write "Dome on Target"(w558) -> ()
                      }
                      frame True {
                        # "Está apontando"
                        n670 = case shown="False" w560 {
                          tunnel: [0 4] -> w561
                          frame False {
                            # "Não verifica\nTrapeira e\nParavento"
                          }
                          frame True {
                            # "Verifica Trapeira e\nParavento"
                            n671 = call "TickTimeout.vi"() -> ("msTick"=w563:u32)  [unwired: 2 in, 2 out]
                            n672 = local write "TimeoutCUP"(w563) -> ()
                            n673 = global write "Global_Telescopio.vi" "T cup"(w563) -> ()
                          }
                        }
                      }
                    }
                  }
                }
              }
              frame 2 {
                w565 = u16 12 items=["Alarme", "Atencao", "Erro", "Ocupado", "TBD", "LCB", "Trapeira", "Paravento", "DomoRap", "DomoCW", "DomoCCW", "TBD", "Em movimento", "TBD"] ("NomeStatus")
                # "Aqui também caberia um Timeout?"
                # "Aguarda parada motor"
                n674 = call "Bit Status CUP.vi"("NomeStatus"=w565) -> ("StatBit"=w567:bool)
                n675 = case shown="False" w567 {
                  tunnel: [1 2] -> w566
                  frame False {
                    # "Motor parado.\nTestar se chegou\nao destino"
                    n676 = call "TickTimeout.vi"() -> ("msTick"=w568:u32)  [unwired: 2 in, 2 out]
                    n677 = local write "TimeoutCUP"(w568) -> ()
                    n678 = global write "Global_Telescopio.vi" "T cup"(w568) -> ()
                  }
                  frame True {
                    # "Ainda movendo...\nAGUARDAR"
                  }
                }
              }
              frame 3 {
                w574 = u16 4 items=["ZERO", "AH", "DEC", "TUBO", "CUP"] ("Controlador")
                # "Trata Timeout"
                n679 = call "TickTimeout.vi"() -> ("msTick"=w571:u32)  [unwired: 2 in, 2 out]
                n680 = local write "TimeoutCUP"(w571) -> ()
                n681 = global write "Global_Telescopio.vi" "T cup"(w571) -> ()
                n682 = call "Monta Comando.vi"("Comando"="PARAR", "Dispositivo"="PROG" ("Comando"), "Controlador"=w574) -> ()  [unwired: 2 in, 5 out]
              }
              frame 4 {
                w577 = u16 7 items=["Alarme", "Atencao", "Erro", "Ocupado", "TBD", "LCB", "Trapeira", "Paravento", "DomoRap", "DomoCW", "DomoCCW", "TBD", "Em movimento", "TBD"] ("NomeStatus")
                # "Verifica Paravento"
                n683 = call "Bit Status CUP.vi"("NomeStatus"=w577) -> ("StatBit"=w581:bool)
                n684 = Not(x=w581) -> (.not. x?=w582:bool)
                n685 = And(x=w582, y="ChkWindDown") -> (x .and. y?=w579:bool)
                n686 = case shown="True" w579 {
                  tunnel: w578 -> [_ w585]
                  tunnel: [6 w584] -> w576
                  frame False {
                    # "Paravento abaixado\nou desabilitado"
                  }
                  frame True {
                    # "Descer Parav."
                    n687 = case shown="False" w585 {
                      tunnel: [5 w590] -> w584
                      frame False {
                        w589 = u16 4 items=["ZERO", "AH", "DEC", "TUBO", "CUP"] ("Controlador")
                        # "Aguardar abaixa/o Parav."
                        # "CLP Pronto"
                        n688 = call "Monta Comando.vi"("Comando"="DESCER", "Dispositivo"="PARAVENTO" ("Comando"), "Controlador"=w589) -> ()  [unwired: 2 in, 5 out]
                      }
                      frame True {
                        # "CLP Busy"
                        n689 = local read "TimeoutCUP"() -> (w592:u32)
                        n690 = call "TickTimeout.vi"("msInicial"=w592, "msTimeout"=u32 5000) -> ("Timeout"=w591:bool)  [unwired: 2 out]
                        n691 = case shown="True" w591 {
                          tunnel: [4 3] -> w590
                          frame False {
                          }
                          frame True {
                          }
                        }
                      }
                    }
                  }
                }
              }
              frame 5 {
                w596 = u16 7 items=["Alarme", "Atencao", "Erro", "Ocupado", "TBD", "LCB", "Trapeira", "Paravento", "DomoRap", "DomoCW", "DomoCCW", "TBD", "Em movimento", "TBD"] ("NomeStatus")
                # "Aqui também caberia um Timeout?"
                # "Também poderia ser testado o bit \"Em movimento\".\nNeste caso o código do \"IF\" deve ser permutado."
                # "Aguarda abaixamento Paravento"
                n692 = call "Bit Status CUP.vi"("NomeStatus"=w596) -> ("StatBit"=w598:bool)
                n693 = case shown="True" w598 {
                  tunnel: [5 6] -> w597
                  frame False {
                    # "Ainda movendo...\nAGUARDAR"
                  }
                  frame True {
                    # "Paravento abaixado."
                  }
                }
              }
              frame 6 {
                w602 = u16 14 items=["Alarme", "Atencao", "Erro", "Ocupado", "Plataforma", "LCB", "Trapeira", "Paravento", "DomoRap", "DomoCW", "DomoCCW", "TBD", "Em movimento", "TrapRUN", "TrapFCH", "TrapABT"] ("NomeStatus")
                # "Verifica Trapeira"
                n694 = call "Bit Status CUP.vi"("NomeStatus"=w602) -> ("StatBit"=w601:bool)
                n695 = And(x=w601, y="ChkOpenShutter") -> (x .and. y?=w604:bool)
                n696 = case shown="True" w604 {
                  tunnel: [0 w610] -> w606
                  tunnel: w603 -> [_ w611]
                  frame False {
                    # "20250910\nTrapeira sempre\ndesabilitada"
                    # "Verificar Paravento"
                    # "Trapeira aberta\nou desabilitada"
                    n697 = call "TickTimeout.vi"() -> ("msTick"=w607:u32)  [unwired: 2 in, 2 out]
                    n698 = local write "TimeoutCUP"(w607) -> ()
                    n699 = global write "Global_Telescopio.vi" "T cup"(w607) -> ()
                    "Dome on Target" <- TRUE
                  }
                  frame True {
                    # "Abrir Trapeira"
                    n700 = case shown="False" w611 {
                      tunnel: [7 w616] -> w610
                      frame False {
                        w615 = u16 4 items=["ZERO", "AH", "DEC", "TUBO", "CUP"] ("Controlador")
                        # "Aguardar abertura Trap."
                        # "CLP Pronto"
